vi "Create AI Group.vi"(8 "error in (no error)":errorcluster, 11 "CVT Tags to Create":T1) -> (0 "error out":errorcluster, 3 "CVT Tags to Create Out":T1)   [LabVIEW 2021, in "CVT.lvlib"]
uses:
  CVT.lvlib
  <vilib>/NI/Current Value Table/Type Defs/File Format.ctl
  <vilib>/NI/Current Value Table/Type Defs/Single Tag.ctl
  <vilib>/NI/Current Value Table/Type Defs/Data Types.ctl
  <vilib>/NI/Current Value Table/Type Defs/Tag Grouping set.ctl
  User Interface/Instrument Address Command.ctl
  User Interface/User Interface.lvlib
  <vilib>/NI/Current Value Table/Current Value Table.lvlib
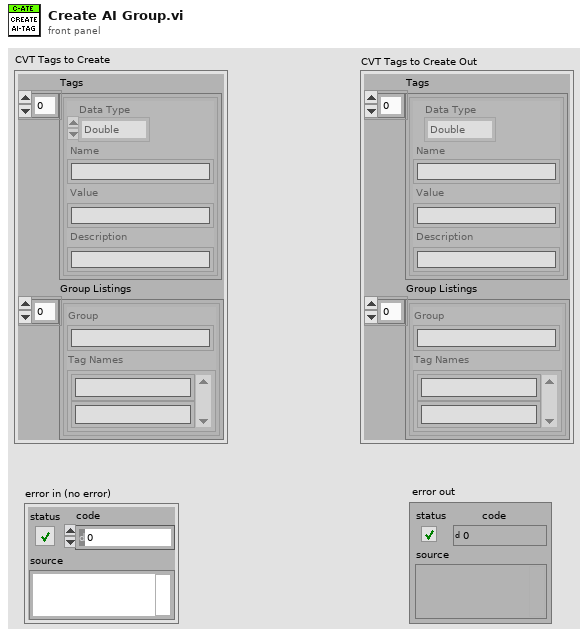
[diagram p1: front panel]
types:
  T1 = typedef "Current Value Table.lvlib/File Format.ctl" = cluster{"Tags":T2[], "Group Listings":T4[]}
  T2 = typedef "Current Value Table.lvlib/Single Tag.ctl" = cluster{"Data Type":T3, "Name":string, "Value":string, "Description":string}
  T3 = typedef "Current Value Table.lvlib/Data Types.ctl" = enum16{"Double", "Single", "I64", "I32", "I16", "I8", "U64", "U32", "U16", "U8", "String", "Boolean", "Array of U8", "Array of U16", "Array of U32", "Array of U64", "Array of I64", "Array of I32", "Array of I16", "Array of I8", "Array of Double", "Array of Single", "Array of Boolean", "Array of String"}
  T4 = typedef "Current Value Table.lvlib/Tag Grouping set.ctl" = cluster{"Group":string, "Tag Names":string[]}
  T5 = typedef "User Interface.lvlib/Instrument Address Command.ctl" = enum16{"Init", "Read", "Write", "Close"}
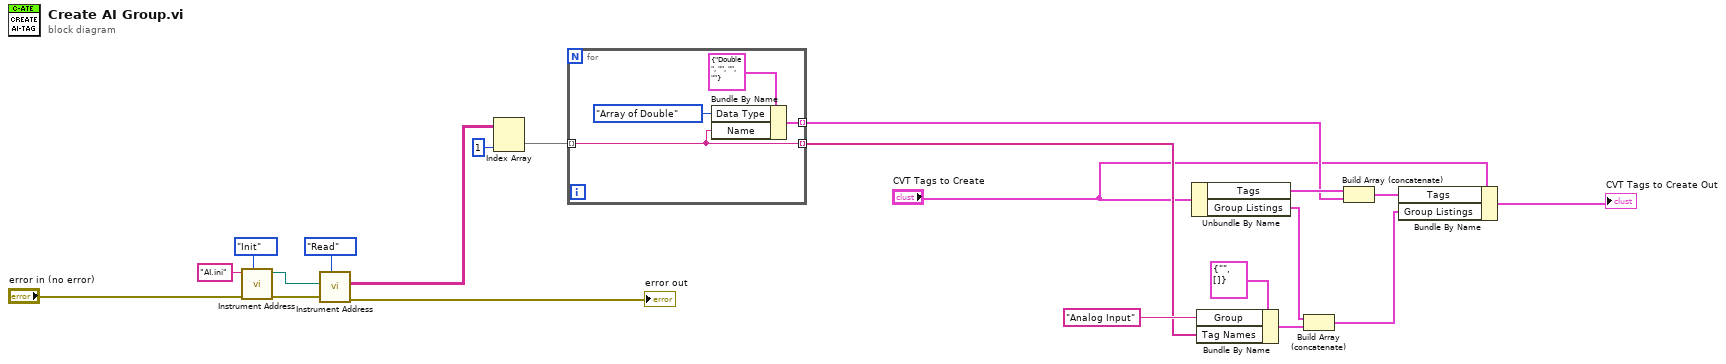
[diagram p0: block diagram]
diagram:
  n1 = call "Instrument Address.vi"("Command"=Instrument_Address_Command."Init", "error in (no error)"="error in (no error)", "name or relative path"="AI.ini") -> ("error out"=w11:errorcluster, "path_out"=w9:path)  [unwired: 6 in, 1 out]
  n2 = call "Instrument Address.vi"("Command"=Instrument_Address_Command."Read", "error in (no error)"=w11, "path_in"=w9) -> ("error out"=→"error out":errorcluster, "Instrument Parameter"=w6:string[][])  [unwired: 6 in, 1 out]
  n3 = Index Array(array=w6, index (col)=1 ("disabled index (col)")) -> (element=w4:string[])  [unwired: 1 in]
  n4 = for {
    tunnel: w4 -> [w24] mode=indexing
    tunnel: [w25] -> w20 mode=indexing
    tunnel: [w24] -> w17 mode=indexing
    n5 = Bundle By Name(cluster=T2 {"Data Type"=enum."Double", "Name"="", "Value"="", "Description"=""} ("element"), "Data Type"=Data_Types."Array of Double", "Name"=w24) -> (w25:T2)
  }
  n6 = Unbundle By Name("CVT Tags to Create") -> ("Tags"=w21:T2[], "Group Listings"=w16:T4[])
  n7 = Bundle By Name(cluster=T4 {"Group"="", "Tag Names"=[]} ("element"), "Group"="Analog Input", "Tag Names"=w17) -> (w15:T4)
  n8 = Build Array (concatenate)(w16, w15) -> (w14:T4[])
  n9 = Build Array (concatenate)(w21, w20) -> (w19:T2[])
  n10 = Bundle By Name(cluster="CVT Tags to Create", "Tags"=w19, "Group Listings"=w14) -> (→"CVT Tags to Create Out":T1)
